vi "Status.vi"(0 "reference in":refnum<class "active object queue.lvclass">, 5 "error in (no error)":errorcluster) -> (14 "reference out":refnum<class "active object queue.lvclass">, 15 "Attribute1":dbl, 16 "Status":bool, 19 "error out":errorcluster)   [LabVIEW 2019, in "active object queue.lvclass"]
uses:
  active object queue.lvclass
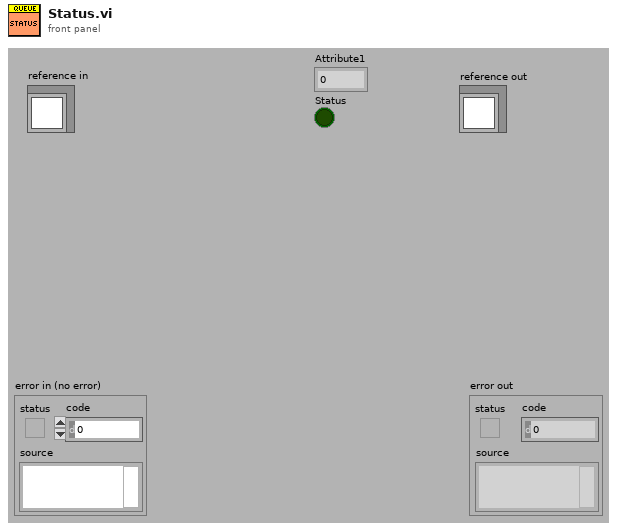
[diagram p1: front panel]
types:
  T1 = typedef "active object queue.lvclass/ObjectAttributes.ctl" = cluster{"Attribute1":dbl, "Status":bool}
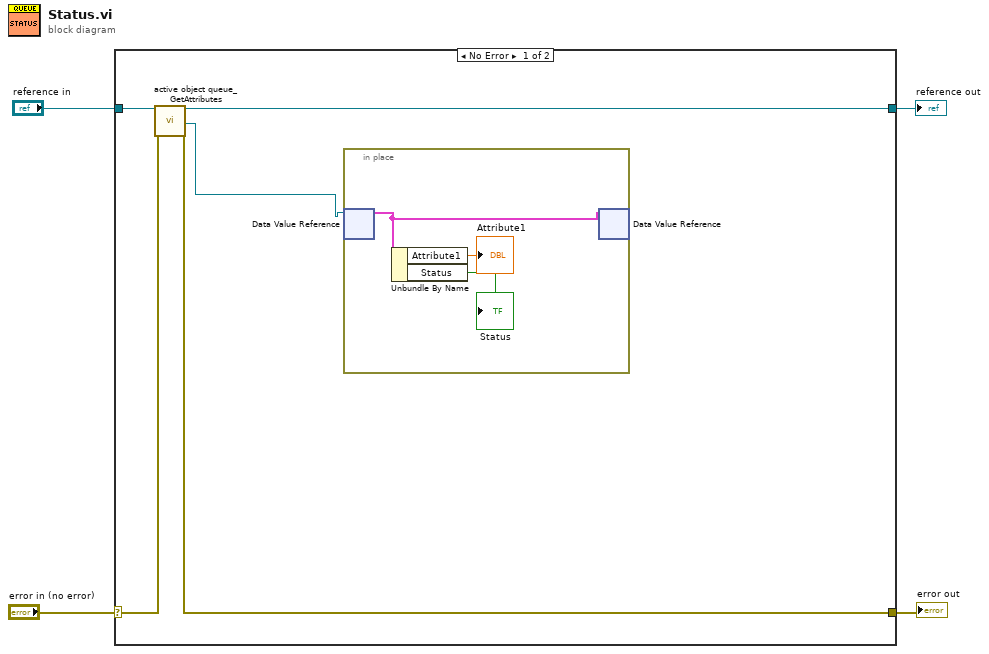
[diagram p0: block diagram]
diagram:
  n1 = case shown="No Error" "error in (no error)" {
    selector: "error in (no error)" -> [w9 w14]
    tunnel: [w8 w14] -> w3
    tunnel: [w6 w13] -> w1
    tunnel: "reference in" -> [w7 w13]
    frame No Error {
      n2 = call "active object queue_GetAttributes.vi"("reference in"=w7, "error in (no error)"=w9) -> ("reference out"=w6:refnum<class "active object queue.lvclass">, "DataRef"=w5:refnum<data-value>, "error out"=w8:errorcluster)  [unwired: 14 in, 1 out]
      n3 = in-place {
        n4 = in-place-dvr #1(w5) -> (w12:T1)  [unwired: 1 out]
        n5 = Unbundle By Name(w12) -> ("Attribute1"=→"Attribute1":dbl, "Status"=→"Status":bool)
        n6 = in-place-dvr #1(w12) -> ()  [unwired: 2 out]
      }
    }
    frame Error {
    }
  }
  "error out" <- w3
  "reference out" <- w1
